vi "Select Robots By Confidence.vi"(11 "robots_blue":T1[](array[typedef]) {"height" format="%+4.3f"; "pixel_y" format="%+4.3f"; "pixel_x" format="%+4.3f"; "orientation" format="%+4.3f"; "y" format="%+4.3f"; "confidence" format="%4.3f"; "x" format="%+4.3f"}) -> (3 "Array":T1[](array[typedef]) {"height" format="%+4.3f"; "pixel_y" format="%+4.3f"; "pixel_x" format="%+4.3f"; "orientation" format="%+4.3f"; "y" format="%+4.3f"; "confidence" format="%4.3f"; "x" format="%+4.3f"})   [LabVIEW 2018]
uses:
  SSL Detection Robot.ctl
  <vilib>/Analysis/Matrix/Datatypes/RealMatrix.ctl
  <vilib>/Analysis/Matrix/NI_Matrix.lvlib
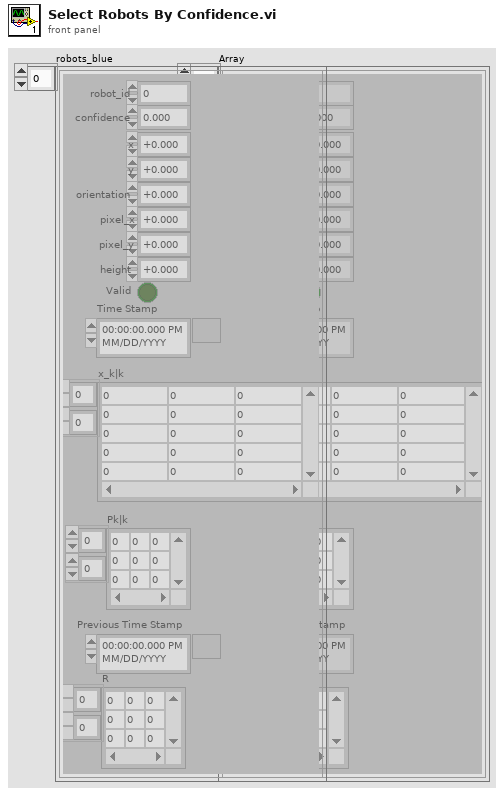
[diagram p1: front panel]
types:
  T1 = typedef "SSL Detection Robot.ctl" = cluster{"x":sgl, "robot_id":u32, "confidence":sgl, "y":sgl, "orientation":sgl, "pixel_x":sgl, "pixel_y":sgl, "height":sgl, "Valid":bool, "Time Stamp":timestamp, "x_k|k":T2, "Pk|k":T2, "Previous Time Stamp":timestamp, "R":T2}
  T2 = typedef "NI_Matrix.lvlib/RealMatrix.ctl" = dbl[][]
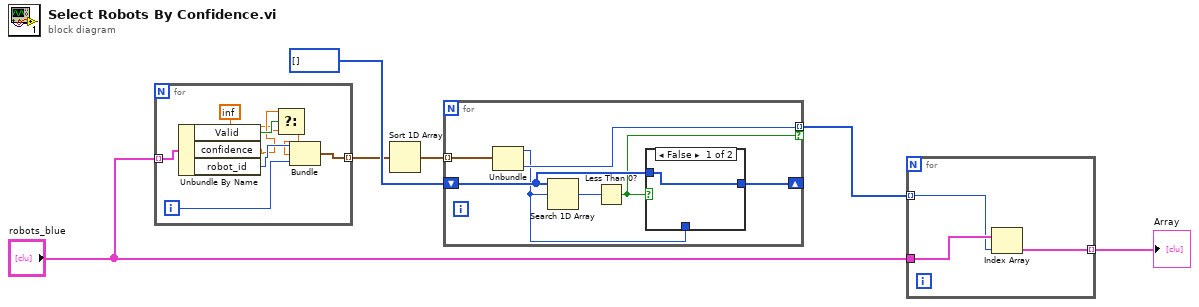
[diagram p0: block diagram]
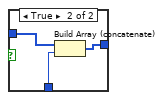
[diagram p2: hidden frame]
diagram:
  n1 = for {
    tunnel: "robots_blue" -> [w14] mode=indexing
    tunnel: [w13] -> w1 mode=indexing
    i -> [w12]
    n2 = Unbundle By Name(w14) -> ("Valid"=w10:bool, "confidence"=w9:sgl, "robot_id"=w11:u32)
    n3 = Select(t=w9, s=w10, f=inf) -> (s? t:f=w8:dbl)
    n4 = Bundle("robot_id"=w11, "confidence"=w8, w12) -> (w13:cluster{"robot_id":u32, "confidence":dbl, i32})  [unwired: 1 in]
  }
  n5 = Sort 1D Array(array=w1) -> (sorted array=w2:cluster{"robot_id":u32, "confidence":dbl, i32}[])
  n6 = for {
    tunnel: w2 -> [w16] mode=indexing
    shift-right: [w19] -> _
    shift-left: i32[] [] -> [w20]
    tunnel: [w18] -> w4 mode=indexing if=w17
    n7 = Unbundle(w16) -> ("robot_id"=w15:u32, w18:i32)  [unwired: 1 out]
    n8 = Search 1D Array(1D array=w20, element=w15) -> (index of element=w21:i32)  [unwired: 1 in]
    n9 = Less Than 0?(x=w21) -> (x < 0?=w17:bool)
    n10 = case shown="False" w17 {
      tunnel: w20 -> [w22 w25]
      tunnel: [w22 w24] -> w19
      tunnel: w15 -> [_ w23]
      frame False {
      }
      frame True {
        n11 = Build Array (concatenate)(w25, w23) -> (w24:u32[])
      }
    }
  }
  n12 = for {
    tunnel: w4 -> [w26] mode=indexing
    tunnel: "robots_blue" -> [w28]
    tunnel: [w27] -> w6 mode=indexing
    n13 = Index Array(array=w28, index=w26) -> (element=w27:T1)
  }
  "Array" <- w6
